vi "SetGlobalWebServiceEnableFlag.vi"(8 "error in (no error)":errorcluster) -> (0 "error out":errorcluster)   [LabVIEW 2017]
uses:
  <vilib>/addons/InsightCM/Utilities/GlobalConfiguration/GlobalConfiguration.lvlib
  <vilib>/addons/InsightCM/Utilities/PropertyHelpers/PropertyHelpers.lvlib
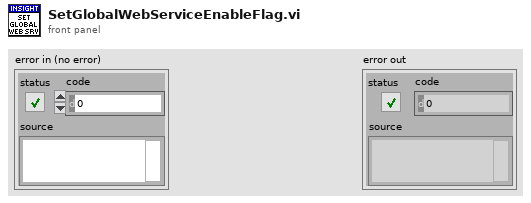
[diagram p1: front panel]
types:
  T1 = typedef "SectionKeyValues.ctl" = cluster{"Section":string, "KeyValues":T2[]}
  T2 = typedef "KeyValuePair.ctl" = cluster{"Key":string, "Value":string}
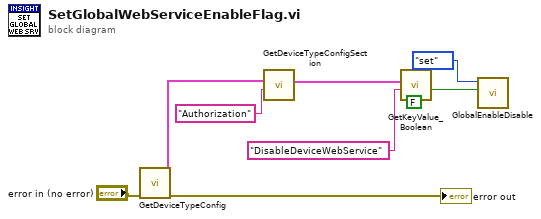
[diagram p0: block diagram]
diagram:
  n1 = call <vilib>:"GetDeviceTypeConfig.vi"("error in (no error)"="error in (no error)") -> ("error out"=→"error out":errorcluster, "key values"=w9:T1[])  [unwired: 8 in, 1 out]
  n2 = call <vilib>:"GetDeviceTypeConfigSection.vi"("key"="Authorization", "key values"=w9) -> ("key value pairs out"=w7:T2[])  [unwired: 8 in, 1 out]
  n3 = call <vilib>:"GetKeyValue_Boolean.vi"("default value"=FALSE, "key"="DisableDeviceWebService", "key value pairs"=w7) -> ("value"=w2:bool)  [unwired: 6 in, 2 out]
  n4 = call "GlobalEnableDisable.vi"("DisableDeviceWebService"=w2, "action"=enum16{"init", "set", "get"}."set") -> ()  [unwired: 9 in, 1 out]
